vi "Set Server Address.vi"(10 "Server Address":string, 11 "OOP Server in":refnum<class "ctet_mux.lvclass">) -> (3 "OOP Server out":refnum<class "ctet_mux.lvclass">)   [LabVIEW 2019, in "ctet_mux.lvlib" / "ctet_mux.lvclass"]
uses:
  ctet_mux.lvclass
  ctet_mux.lvclass/ctet_mux.ctl
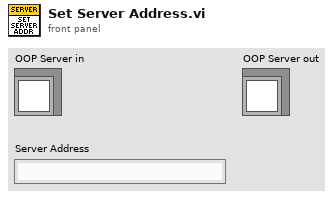
[diagram p1: front panel]
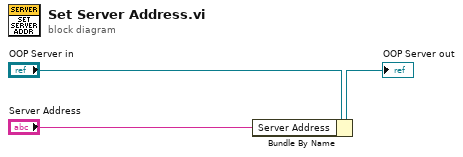
[diagram p0: block diagram]
diagram:
  n1 = Bundle By Name(cluster="OOP Server in", "Server Address"="Server Address") -> (→"OOP Server out":refnum<class "ctet_mux.lvclass">)
